vi "Update Timer Display.vi"(8 "error in (no error)":errorcluster, 9 "Current Time":dbl, 10 "Starting Time":dbl, 11 "MC Prompt in":refnum<class "MC Prompt.lvclass">) -> (0 "error out":errorcluster, 3 "MC Prompt out":refnum<class "MC Prompt.lvclass">)   [LabVIEW 2021, in "MC Prompt.lvlib" / "MC Prompt.lvclass"]
uses:
  MC Prompt.lvclass
  MC Prompt.lvclass/MC Prompt.ctl
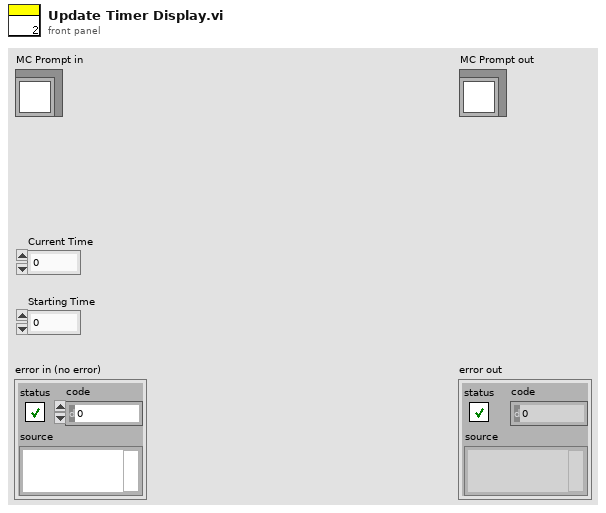
[diagram p1: front panel]
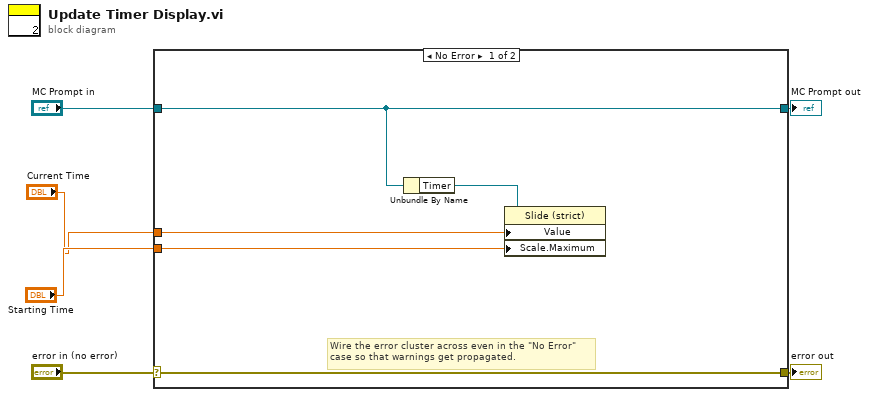
[diagram p0: block diagram]
diagram:
  n1 = case shown="No Error" "error in (no error)" {
    selector: "error in (no error)" -> [w11 w13]
    tunnel: [w11 w13] -> w5
    tunnel: [w9 w12] -> w3
    tunnel: "MC Prompt in" -> [w9 w12]
    tunnel: "Starting Time" -> [w8 _]
    tunnel: "Current Time" -> [w7 _]
    frame No Error {
      # "Wire the error cluster across even in the \"No Error\"\ncase so that warnings get propagated."
      n2 = Unbundle By Name(w9) -> ("Timer"=w10:refnum<vi>)
      n3 = property class="Slide (strict)"(reference=w10, "Value"=w7, "Scale.Maximum"=w8) -> ()  [unwired: 1 in, 2 out]
    }
    frame Error {
    }
  }
  "error out" <- w5
  "MC Prompt out" <- w3
